vi "Main.vi"() -> ()   [LabVIEW 2016]
uses:
  pressure_cluster.ctl
  adsorbed_cluster.ctl
  EOS.ctl
  auxiliary_cluster.ctl
panel:
  in  "?":T1(tab)
  in  "Leak Rate Calibration":path
  in  "Rig Volume Calibration":path
  in  "Sample Density Calibration":path
  in  "Experimental Folder":path
  in  "Absolute adsorption":enum16{"Micropore_filling", "Surface_coverage"}(ring)
  in  "EOS":T2 items=["Ideal", "CH4_van_der_Waal", "CH4_Redlich_Kwong", "CO2_van_der_Waal", "CO2_Redlich_Kwong", ""]
  in  "Sample Weight (g)":dbl
  in  "Start":bool
  in  "Stop":bool
  in  "Tab Control":enum32{"Isotherm", "Equilirium Pressures"}(tab)
  out "XY Graph":cluster{"X":dbl, "Y":dbl}[](graph)
  in  "Pressure Calibration":enum32{"Previous Pressure", "Initial Pressure"}(tab)
  out "Starting in":dbl format="%#_1g"
  in  "Start Button":bool
  in  "?":T3(tab)
  out "P Chart":dbl(graph)
  out "n Chart":T4(graph)
  in  "?":enum32{"Auxiliary Data", "Last Reading"}(tab)
  in  "Rate of sorption threshold":dbl
  in  "Auxiliary Data":T5 {"Absolute adsorption" items=["Micropore_filling", "Surface_coverage"]; "EOS" items=["Ideal", "CH4_van_der_Waal", "CH4_Redlich_Kwong", "CO2_van_der_Waal", "CO2_Redlich_Kwong", ""]}
  in  "Max Duration (hrs)":dbl(slide)=6.0 min=2.0 max=24.0 step=1.0 scale=2.0..24.0
  in  "Frequency (secs)":u32=10 min=1 max=600 step=1
  in  "Stop Button":bool
  out "z":dbl
  out "rho_bulk (g/cc)":dbl
  out "Rate of sorption":bool
  out "Last Reading":T6 {"Temperature" scale=0.0..400.0; "Pressure (barg)" scale=0.0..70.0}
  out "Duration (secs)":dbl(slide) scale=0.0..21600.0
  # "Manometric Adsorption Measurement Rig"
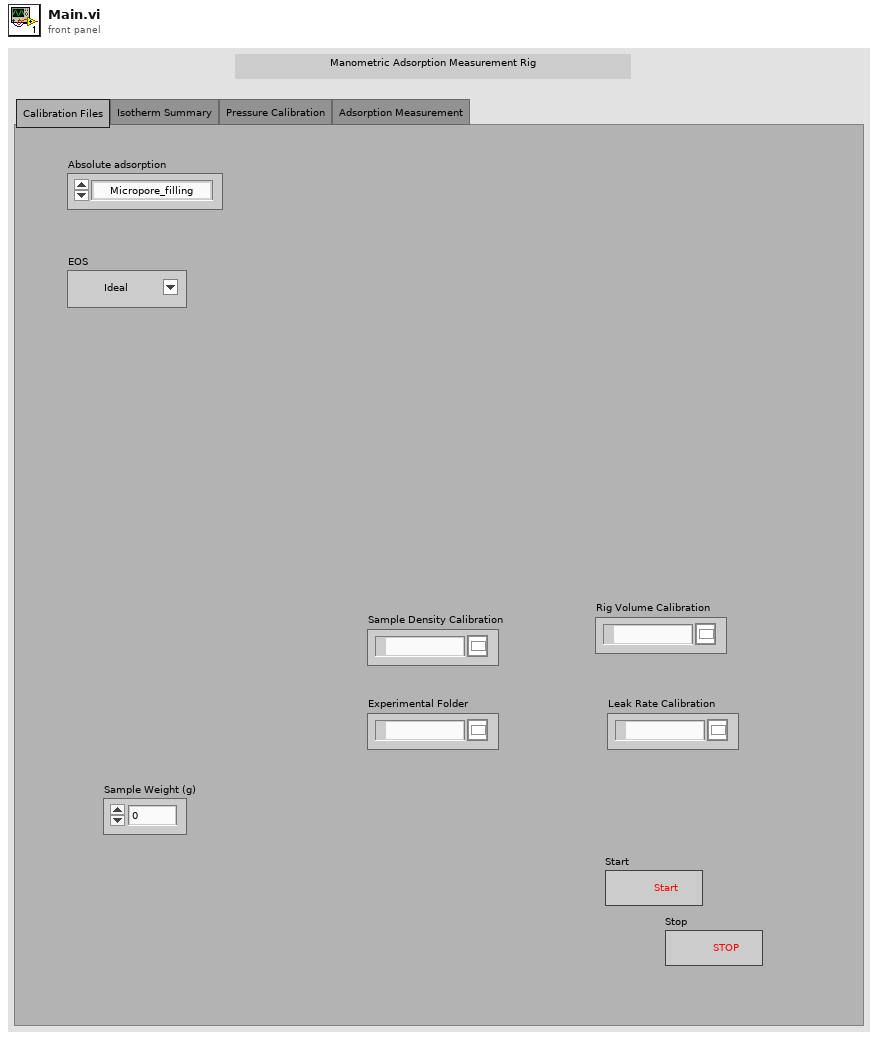
[diagram p1: front panel]
types:
  T1 = enum32{"Calibration Files", "Isotherm Summary", "Pressure Calibration", "Adsorption Measurement"}
  T2 = typedef "EOS.ctl" = u16
  T3 = enum32{"Pressure ", "Temperature", "Amount Adsorbed", "Rate of Sorption"}
  T4 = cluster{"n_excess (mmol/g)":dbl, "n_abs (mmol/g)":dbl}
  T5 = typedef "auxiliary_cluster.ctl" = cluster{"Pi (barg)":dbl, "Pfp (barg)":dbl, "Vr (ml)":dbl, "w (g)":dbl, "EOS":T2, "rho_ads (g/ml)":dbl, "MW (g/mol)":dbl, "Vv (ml)":dbl, "Absolute adsorption":u16}
  T6 = typedef "adsorbed_cluster.ctl" = cluster{"Time":timestamp, "Pressure (barg)":dbl, "n_excess (mmol/g)":dbl, "n_abs (mmol/g)":dbl, "Temperature":dbl}
  T7 = cluster{"n_excess (mmol/g)":dbl, "n_abs (mmol/g)":dbl}[]
  T8 = typedef "pressure_cluster.ctl" = cluster{"Time":timestamp, "Pressure (barg)":dbl, "T (K)":dbl}
  T9 = enum8{"Enabled", "Disabled", "Disabled and Grayed Out"}
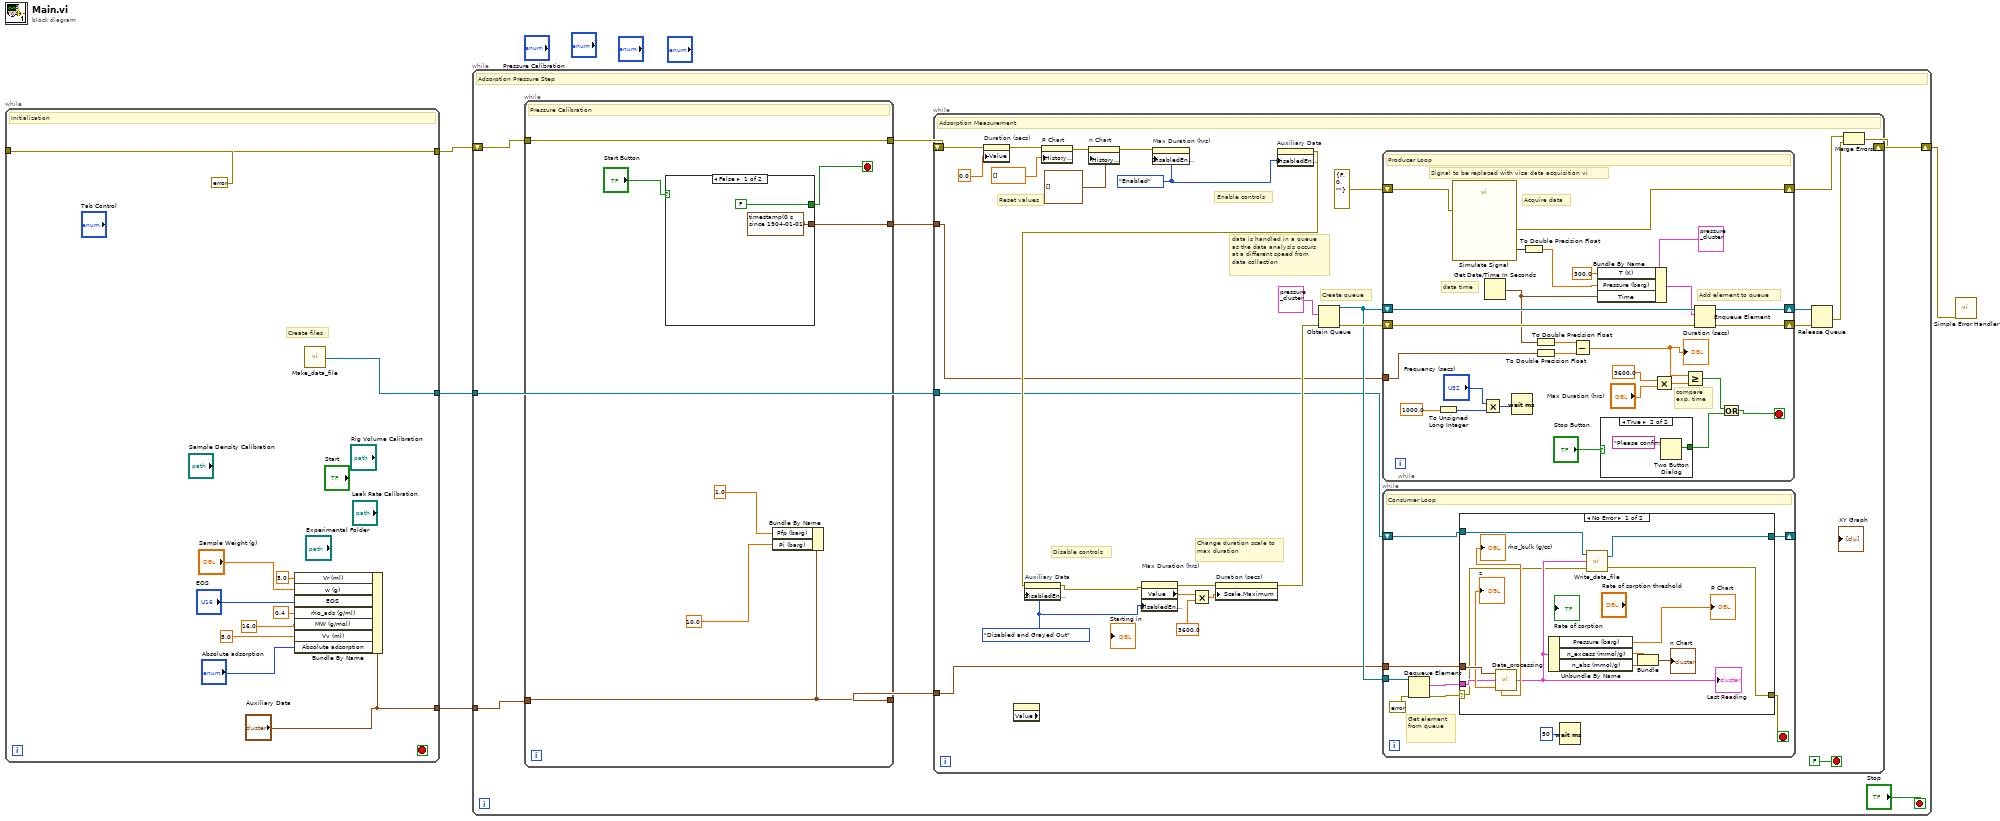
[diagram p0: block diagram]
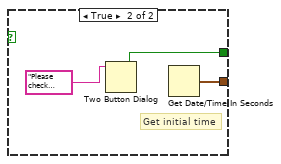
[diagram p2: hidden frame]
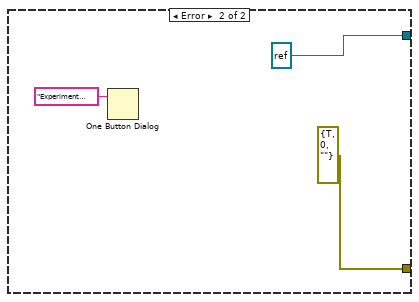
[diagram p3: hidden frame]
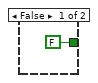
[diagram p4: hidden frame]
diagram:
  n1 = while {
    tunnel: errorcluster {"status"=FALSE, "code"=0, "source"=""} ("error in (no error)") -> [w15]
    tunnel: [w15] -> w3
    tunnel: ["Auxiliary Data"] -> w2
    tunnel: [w6] -> w1
    stop <- _ stop-if-true
    # "Create files"
    # "Initialization"
    n2 = Bundle By Name(cluster="Auxiliary Data", "Vr (ml)"=5.0, "w (g)"="Sample Weight (g)", "EOS"="EOS", "rho_ads (g/ml)"=0.4, "MW (g/mol)"=16.0, "Vv (ml)"=5.0, "Absolute adsorption"="Absolute adsorption") -> ()  [unwired: 1 out]
    n3 = call "Make_data_file.vi"() -> ("File Refnum"=w6:refnum<file>)  [unwired: 1 in]
  }
  n4 = while {
    tunnel: w2 -> [w19]
    tunnel: w1 -> [w18]
    shift-right: [w23] -> w5
    shift-left: w3 -> [w20]
    stop <- "Stop" stop-if-true
    # "Adsorption Pressure Step"
    n5 = while {
      tunnel: [w29] -> w22
      tunnel: w20 -> [w30]
      tunnel: [w30] -> w21
      tunnel: w19 -> [w29]
      tunnel: [w26] -> w17
      stop <- w25 stop-if-true
      # "Pressure Calibration"
      n6 = case shown="False" "Start Button" {
        tunnel: [FALSE ("T button?") w34] -> w25
        tunnel: [timestamp(0 s since 1904-01-01) ("seconds since 1Jan1904") w35] -> w26
        frame False {
        }
        frame True {
          # "Get initial time"
          n7 = Two Button Dialog(message="Please check auxiliary data, file name, and max. duration and cofirm if you want to proceed.") -> (T button?=w34:bool)  [unwired: 2 in]
          n8 = Get Date/Time In Seconds() -> (seconds since 1Jan1904=w35:timestamp)
        }
      }
      n9 = Bundle By Name(cluster=w29, "Pfp (barg)"=1.0, "Pi (barg)"=10.0) -> ()  [unwired: 1 out]
    }
    n10 = while {
      shift-right: [w56] -> w23
      shift-left: w21 -> [w53]
      tunnel: w22 -> [w39]
      tunnel: w18 -> [w38]
      tunnel: w17 -> [w37]
      stop <- FALSE stop-if-true
      w44 = T9."Disabled and Grayed Out" ("Disabled")
      w45 = T9."Enabled" ("Disabled")
      # "data is handled in a queue \nas the data analysis occurs \nat a different speed from \ndata collection"
      # "Disable controls"
      # "Enable controls"
      # "Reset values"
      # "Create queue"
      # "Change duration scale to max duration"
      # "Adsorption Measurement"
      n11 = property on="Duration (secs)" class="Slide (strict)"(error in=w53, "Value"=0.0 ("Duration (hrs)")) -> (error out=w52:errorcluster)  [unwired: 1 in, 1 out]
      n12 = property class="TabCtl (strict)" props=["Value"]() -> ()  [unwired: 2 in, 3 out]
      n13 = property on="P Chart" class="WFChart (strict)"(error in=w52, "History Data"=dbl[] []) -> (error out=w49:errorcluster)  [unwired: 1 in, 1 out]
      n14 = property on="n Chart" class="WFChart (strict)"(error in=w49, "History Data"=T7 []) -> (error out=w46:errorcluster)  [unwired: 1 in, 1 out]
      n15 = property on="Max Duration (hrs)" class="Slide (strict)"(error in=w46, "DisabledEnum"=w45) -> ()  [unwired: 1 in, 2 out]
      n16 = property on="Auxiliary Data" class="Clust (strict)"("DisabledEnum"=w45) -> (error out=w47:errorcluster)  [unwired: 2 in, 1 out]
      n17 = property on="Auxiliary Data" class="Clust (strict)"(error in=w47, "DisabledEnum"=w44) -> (error out=w36:errorcluster)  [unwired: 1 in, 1 out]
      n18 = property on="Max Duration (hrs)" class="Slide (strict)"(error in=w36, "DisabledEnum"=w44) -> (error out=w55:errorcluster, "Value"=w41:dbl)  [unwired: 1 in, 1 out]
      n19 = Multiply(x=w41, y=3600.0) -> (x*y=w42:dbl)
      n20 = property on="Duration (secs)" class="Slide (strict)"(error in=w55, "Scale.Maximum"=w42) -> (error out=w43:errorcluster)  [unwired: 1 in, 1 out]
      n21 = Obtain Queue(element data type=T8 {"Time"=timestamp(0 s since 1904-01-01), "Pressure (barg)"=0.0, "T (K)"=0.0} ("Presssure"), error in (no error)=w43) -> (queue out=w59:refnum<queue>, error out=w64:errorcluster)  [unwired: 3 in, 1 out]
      n22 = while {
        shift-right: [w108] -> w60
        shift-left: w59 -> [w109]
        shift-right: [w106] -> w61
        shift-left: w64 -> [w107]
        shift-right: [w114] -> w57
        shift-left: errorcluster {"status"=FALSE, "code"=0, "source"=""} ("error out") -> [w115]
        tunnel: w37 -> [w103]
        stop <- w101 stop-if-true
        # "Add element to queue"
        # "Acquire data"
        # "data time"
        # "compare exp. time"
        # "Signal to be replaced with visa data acquisition vi"
        # "Producer Loop"
        n23 = To Unsigned Long Integer(number=1000.0 ("y")) -> (unsigned 32bit integer=w110:u32)
        n24 = call "Simulate Signal"("error in (no error)"=w115) -> ("Triangle with Uniform Noise"=w116:dynamicdata, "error out"=w114:errorcluster)  [unwired: 13 in]
        n25 = Multiply(x="Frequency (secs)", y=w110) -> (x*y=w112:u32)
        n26 = Get Date/Time In Seconds() -> (seconds since 1Jan1904=w99:timestamp)
        n27 = Wait (ms)(milliseconds to wait=w112) -> ()  [unwired: 1 out]
        n28 = To Double Precision Float(number=w116) -> (double precision float=w97:dbl)
        n29 = To Double Precision Float(number=w99) -> (double precision float=w104:dbl)
        n30 = To Double Precision Float(number=w103) -> (double precision float=w105:dbl)
        n31 = Subtract(x=w104, y=w105) -> (x-y=w91:dbl)
        "Duration (secs)" <- w91
        n32 = Bundle By Name(cluster=T8 {"Time"=timestamp(0 s since 1904-01-01), "Pressure (barg)"=0.0, "T (K)"=0.0} ("Presssure"), "T (K)"=300.0, "Pressure (barg)"=w97, "Time"=w99) -> (w98:T8)
        n33 = case shown="True" "Stop Button" {
          tunnel: [FALSE ("T button?") w119] -> w96
          frame False {
          }
          frame True {
            n34 = Two Button Dialog(message="Please confirm if you want to stop the experiment, before max. duration.") -> (T button?=w119:bool)  [unwired: 2 in]
          }
        }
        n35 = Multiply(x=3600.0 ("y"), y="Max Duration (hrs)") -> (x*y=w92:dbl)
        n36 = Greater Or Equal?(x=w91, y=w92) -> (x >= y?=w102:bool)
        n37 = Enqueue Element(queue=w109, element=w98, error in (no error)=w107) -> (queue out=w108:refnum<queue>, error out=w106:errorcluster)  [unwired: 1 in, 1 out]
        n38 = Or(x=w102, y=w96) -> (x .or. y?=w101:bool)
      }
      n39 = while {
        tunnel: w39 -> [w72]
        tunnel: w59 -> [w68]
        shift-right: [w65] -> _
        shift-left: w38 -> [w66]
        stop <- w73 stop-if-true
        # "Get element from queue"
        # "Consumer Loop"
        n40 = Dequeue Element(queue=w68, error in (no error)=errorcluster {"status"=FALSE, "code"=0, "source"=""}) -> (element=w70:T8, error out=w69:errorcluster)  [unwired: 1 in, 2 out]
        n41 = case shown="No Error" w69 {
          selector: w69 -> [w75 _]
          tunnel: w70 -> [w79 _]
          tunnel: [w74 errorcluster {"status"=TRUE, "code"=0, "source"=""} ("error IO")] -> w73
          tunnel: w72 -> [w85 _]
          tunnel: w66 -> [w78 _]
          tunnel: [w76 refnum<file> refnum ("output file refnum")] -> w65
          frame No Error {
            n42 = call "Data_processing.vi"("Presssure"=w79, "Auxiliary"=w85) -> ("z"=→"z":dbl, "Latest Data"=w77:T6, "rho_bulk"=→"rho_bulk (g/cc)":dbl)  [unwired: 1 in]
            "Last Reading" <- w77
            n43 = Unbundle By Name(w77) -> ("Pressure (barg)"=→"P Chart":dbl, "n_excess (mmol/g)"=w82:dbl, "n_abs (mmol/g)"=w81:dbl)
            n44 = call "Write_data_file.vi"("error in"=w75, "Latest_Data"=w77, "Input file refnum"=w78) -> ("error out"=w74:errorcluster, "output file refnum"=w76:refnum<file>)
            n45 = Bundle("n_excess (mmol/g)"=w82, "n_abs (mmol/g)"=w81) -> (→"n Chart":T4)  [unwired: 1 in]
          }
          frame Error {
            n46 = One Button Dialog(message="Experiment complete.") -> ()  [unwired: 1 in, 1 out]
          }
        }
        n47 = Wait (ms)(milliseconds to wait=u32 50) -> ()  [unwired: 1 out]
      }
      n48 = Release Queue(queue=w60, error in (no error)=w61) -> (error out=w58:errorcluster)  [unwired: 1 in, 2 out]
      n49 = Merge Errors(w57, w58) -> (w56:errorcluster)
    }
  }
  n50 = call <vilib>:"Simple Error Handler.vi"("error in (no error)"=w5) -> ()  [unwired: 4 in, 5 out]
